vi "Get Bounds and Position.vi"(8 "error in (no error)":errorcluster, 11 "ViewableActor in":refnum<class "ViewableActor.lvclass">) -> (0 "error out":errorcluster, 1 "Windows Bounds":T2, 2 "Panel Bounds":T3, 3 "ViewableActor out":refnum<class "ViewableActor.lvclass">, 4 "Panel Position":T1)   [LabVIEW 2020, in "ViewableActor.lvlib" / "ViewableActor.lvclass"]
uses:
  ViewableActor.lvclass
  <vilib>/Utility/miscctls.llb/LVBoundsTypeDef.ctl
  <vilib>/Utility/miscctls.llb/LVRectTypeDef.ctl
  <vilib>/Utility/miscctls.llb/LVPositionTypeDef.ctl
  ViewableActor.lvclass/ViewableActor.ctl
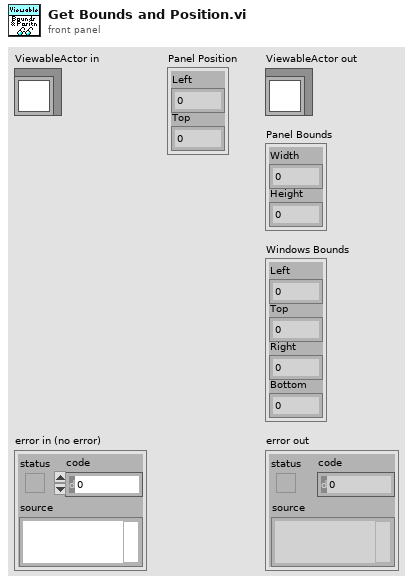
[diagram p1: front panel]
types:
  T1 = typedef "LVPositionTypeDef.ctl" = cluster{"Left":i32, "Top":i32}
  T2 = typedef "LVRectTypeDef.ctl" = cluster{"Left":i16, "Top":i16, "Right":i16, "Bottom":i16}
  T3 = typedef "LVBoundsTypeDef.ctl" = cluster{"Width":u32, "Height":u32}
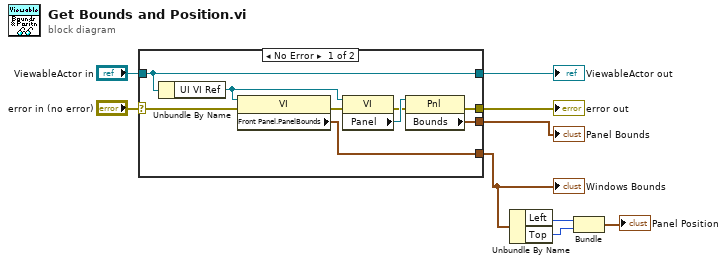
[diagram p0: block diagram]
diagram:
  n1 = case shown="No Error" "error in (no error)" {
    selector: "error in (no error)" -> [w11 w20]
    tunnel: [w10 w20] -> w8
    tunnel: [w18 w19] -> w6
    tunnel: "ViewableActor in" -> [w18 w19]
    tunnel: [w16 _] -> w5
    tunnel: [w14 _] -> w4
    frame No Error {
      n2 = Unbundle By Name(w18) -> ("UI VI Ref"=w15:refnum<vi>)
      n3 = property class="VI"(reference=w15, error in=w11) -> (error out=w13:errorcluster, "Front Panel.PanelBounds"=w14:T2)  [unwired: 1 out]
      n4 = property class="VI"(reference=w15, error in=w13) -> (error out=w12:errorcluster, "Panel"=w17:refnum<vi>)  [unwired: 1 out]
      n5 = property class="Pnl"(reference=w17, error in=w12) -> (error out=w10:errorcluster, "Bounds"=w16:T3)  [unwired: 1 out]
    }
    frame Error {
    }
  }
  "error out" <- w8
  "ViewableActor out" <- w6
  "Panel Bounds" <- w5
  "Windows Bounds" <- w4
  n6 = Unbundle By Name(w4) -> ("Left"=w3:i16, "Top"=w2:i16)
  n7 = Bundle("Left"=w3, "Top"=w2) -> (→"Panel Position":cluster{"Left":i16, "Top":i16})  [unwired: 1 in]
